vi "OAT Torsional Vibration (Analog Tacho) (Even-Angle) (1 Ch).vi"(0 "analog tacho signal":waveform(dbl)={"t0"=timestamp(0 s since 1904-01-01), "dt"=0.0, "Y"=[]}, 1 "threshold (auto)":dbl=inf format="%.2f", 2 "pulse/revolution (1)":i32=1 min=1, 3 "hysteresis (0)":dbl format="%.2f", 4 "torsional vibration units":enum16{"RPM", "deg/s", "rad/s"}(ring), 5 "error in (no error)":errorcluster, 6 "missing pulses? (no:F)":bool, 7 "pulse width (2)":i32=2 min=0, 8 "reset? (F)":bool, 9 "slope (Rising)":u16(ring) items=["Rising", "Falling"]) -> (14 "even-angle torsional vibration signal":cluster{"r0":dbl, "dr":dbl, "Y":dbl[]}={"r0"=0.0, "dr"=1.0, "Y"=[]} {"r0" format="%.2p"; "dr" format="%.2p"; "Y" format="%.2f"}, 15 "even-angle channel info":T3={"channel name"="", "description"="", " channel info"={"sensor sensitivity"=1000.0, "engineering units"=1, "dB reference"=1.0, "custom label"="EU", "weighting filter"=0, "pregain"=0.0}} {"channel info"."pregain" format="%.2f"; "channel info"."weighting filter" items=["Linear", "A-weighting", "B-weighting", "C-weighting", "ITU-R 468-4", "Dolby", "CCITT", "C-message", "Wb", "Wc", "Wd", "We", "Wf", "Wh", "Wj", "Wk", "Wm", "AES17 20 kHz lowpass", "AES17 40 kHz lowpass", "AES17 20 kHz highpass", "AES17 40 kHz highpass"]; "channel info"."dB reference" format="%^.1e"; "channel info"."engineering units" items=["custom..."=0, "V"=1, "A"=21, "C"=30, "pC"=31, "s"=32, "-"=29, "Pa"=2, "N"=20, "g"=3, "m/s^2"=4, "m/s"=5, "m"=6, "mm/s"=12, "mm"=13, "micron/s"=14, "micron"=15, "in/s^2"=7, "in/s"=8, "in"=9, "mil/s"=10, "mil"=11, "rad/s^2"=16, "rad/s"=17, "rad"=18, "deg/s^2"=26, "deg/s"=27, "deg"=28, "RPM"=22, "cycle/s^2"=23, "Hz"=24, "cycle"=25, "strain"=19]; "channel info"."sensor sensitivity" format="%#_5f"}, 16 "speed profile":T2 {"speed [RPM]" format="%.2f"; "time [s]" format="%.2f"}, 17 "position info":T1, 18 "unit label":string, 19 "error out":errorcluster)   [LabVIEW 2017, in "SoundVib_Torsional.lvlib"]
doc: "Calculates torsional vibration signals from analog tachometer signals. This VI can return torsional vibration signals as either waveform signals or even-angle signals. Wire data to the <B>analog tacho signal</B> input to determine the polymorphic instance to use or manually select the instance."
uses:
  <vilib>/addons/Sound and Vibration/Order Analysis/Torsional Vibration/SoundVib_Torsional.lvlib
  <vilib>/addons/_NISVFA/_Shared subVIs/Controls/svc_Resampled Channel Info.ctl
  <vilib>/addons/_NISVFA/_Shared subVIs/Controls/svc_Channel Info.ctl
  <vilib>/addons/_NISVFA/_Shared subVIs/Controls/svc_Engineering Units Text Ring.ctl
  <vilib>/addons/_NISVFA/_Shared subVIs/Controls/svc_Weighting Filter Text Ring.ctl
  <vilib>/addons/Sound and Vibration/Order Analysis/Tach Process/SubVIs/speed profile.ctl
  <vilib>/addons/Sound and Vibration/Order Analysis/Misc/OAT Position Info.ctl
  <vilib>/addons/_NISVFA/_Shared subVIs/Common/svc_Check for Waveform Parameter Continuity (no state).vi
  <vilib>/addons/_NISVFA/_Shared subVIs/Common/svc_Get SV Channel Info.vi
  <vilib>/addons/_NISVFA/_Shared subVIs/Common/svc_Engineering Units to Unit Label.vi
  <vilib>/addons/_NISVFA/_Shared subVIs/Common/svc_Unit Label to Engineering Units.vi
  <vilib>/addons/Sound and Vibration/Order Analysis/Tach Process/SoundVib_TachProcess.lvlib
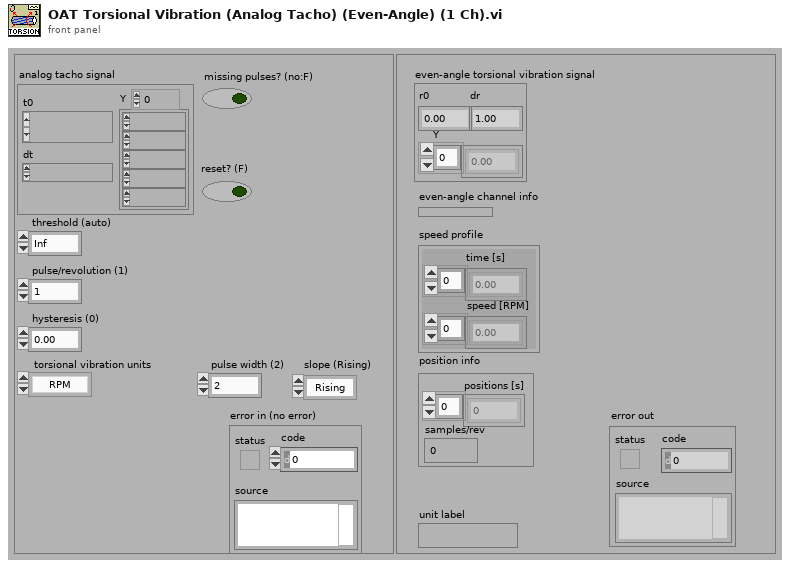
[diagram p1: front panel]
types:
  T1 = typedef "OAT Position Info.ctl" = cluster{"positions [s]":dbl[], "samples/rev":dbl}
  T2 = typedef "SoundVib_TachProcess.lvlib/speed profile.ctl" = cluster{"time [s]":dbl[], "speed [RPM]":dbl[]}
  T3 = typedef "svc_Resampled Channel Info.ctl" = cluster{"channel name":string, "description":string, " channel info":T4}
  T4 = typedef "svc_Channel Info.ctl" = cluster{"sensor sensitivity":dbl, "engineering units":T5, "dB reference":dbl, "custom label":string, "weighting filter":T6, "pregain":dbl}
  T5 = typedef "svc_Engineering Units Text Ring.ctl" = u16
  T6 = typedef "svc_Weighting Filter Text Ring.ctl" = u16
  T7 = cluster{"dt":bool, "t0 continuity":bool, "array length":bool, "channel info":bool, "name":bool}
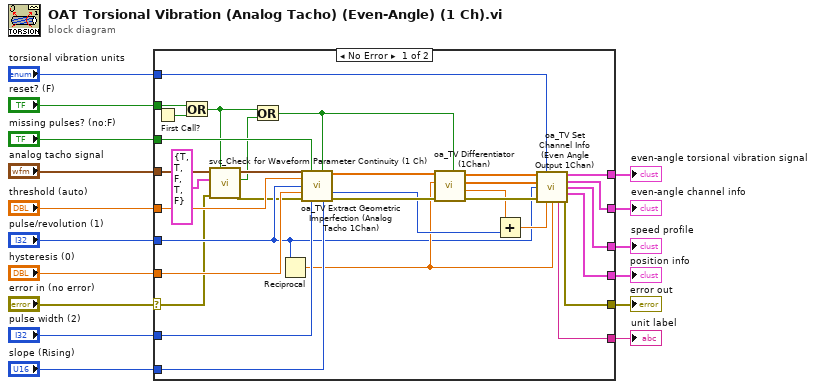
[diagram p0: block diagram]
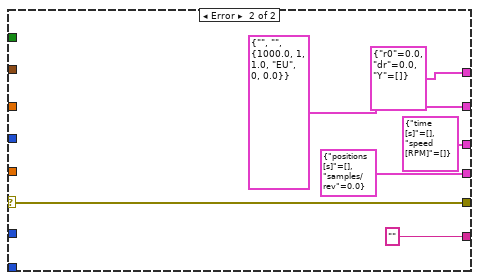
[diagram p2: hidden frame]
diagram:
  n1 = case shown="No Error" "error in (no error)" {
    selector: "error in (no error)" -> [w22 w52]
    tunnel: "analog tacho signal" -> [w48 _]
    tunnel: "threshold (auto)" -> [w47 _]
    tunnel: "pulse/revolution (1)" -> [w25 _]
    tunnel: "pulse width (2)" -> [w46 _]
    tunnel: "slope (Rising)" -> [w35 _]
    tunnel: "hysteresis (0)" -> [w45 _]
    tunnel: [w40 w52] -> w11
    tunnel: "reset? (F)" -> [w43 _]
    tunnel: "torsional vibration units" -> [w32 _]
    tunnel: [w36 T3 {"channel name"="", "description"="", " channel info"={"sensor sensitivity"=1000.0, "engineering units"=1, "dB reference"=1.0, "custom label"="EU", "weighting filter"=0, "pregain"=0.0}} ("even-angle channel info")] -> w7
    tunnel: [w37 cluster{"r0":dbl, "dr":dbl, "Y":dbl[]} {"r0"=0.0, "dr"=0.0, "Y"=[]} ("even-angle torsional vibration")] -> w6
    tunnel: [w31 T1 {"positions [s]"=[], "samples/rev"=0.0} ("speed position info")] -> w2
    tunnel: [w29 T2 {"time [s]"=[], "speed [RPM]"=[]} ("speed profile")] -> w4
    tunnel: "missing pulses? (no:F)" -> [w28 _]
    tunnel: [w26 "" ("unit label")] -> w1
    frame No Error {
      n2 = First Call?() -> (First Call?: T/F=w44:bool)
      n3 = Or(x=w43, y=w44) -> (x .or. y?=w19:bool)
      n4 = call <vilib>:"svc_Check for Waveform Parameter Continuity (1 Ch).vi"("restart averaging (F)"=w19, "error in (no error)"=w22, "checks for channel parameter change"=T7 {"dt"=TRUE, "t0 continuity"=TRUE, "array length"=FALSE, "channel info"=TRUE, "name"=FALSE}, "scaled signal [EU]"=w48) -> ("error out"=w21:errorcluster, "waveform parameter changed"=w18:bool, "dup scaled signal [EU]"=w23:waveform(dbl))  [unwired: 2 in, 3 out]
      n5 = Or(x=w19, y=w18) -> (x .or. y?=w20:bool)
      n6 = Reciprocal(x=w25) -> (1/x=w27:dbl)
      n7 = call <vilib>:"oa_TV Extract Geometric Imperfection (Analog Tacho 1Chan).vi"("analog tacho signal"=w23, "missing pulses? (no:F)"=w28, "reset? (F)"=w20, "threshold (auto)"=w47, "pulse/revolution"=w25, "hysteresis(0)"=w45, "error in (no error)"=w21, "pulse width (2)"=w46, "slope (Rising)"=w35) -> ("pulse positions"=w42:dbl[], "revulotion index"=w33:i32, "error out"=w34:errorcluster)  [unwired: 3 in, 1 out]
      n8 = call <vilib>:"oa_TV Differentiator (1Chan).vi"("reset? (True)"=w20, "error in (no error)"=w34, "deltaX"=w27, "Y[n]"=w42) -> ("error out"=w41:errorcluster, "Delay"=w24:dbl, "X[n]"=w30:dbl[], "dY[n]/dX[n]"=w38:dbl[])  [unwired: 4 in]
      n9 = Add(x=w24, y=w33) -> (x+y=w39:dbl)
      n10 = call <vilib>:"oa_TV Set Channel Info (Even Angle Output 1Chan).vi"("seconds/rev"=w38, "torisional vibration unit (RPM)"=w32, "pulse position"=w30, "pulse/revolution (1)"=w25, "error in (no error)"=w41, "r0"=w39, "dr"=w27) -> ("even-angle torsional vibration"=w37:cluster{"r0":dbl, "dr":dbl, "Y":dbl[]}, "even-angle channel info"=w36:T3, "speed profile"=w29:T2, "position info"=w31:T1, "unit label"=w26:string, "error out"=w40:errorcluster)  [unwired: 3 in]
    }
    frame Error {
    }
  }
  "error out" <- w11
  "even-angle torsional vibration signal" <- w6
  "even-angle channel info" <- w7
  "speed profile" <- w4
  "position info" <- w2
  "unit label" <- w1
